vi "16 pulses TX.vi"(7 "reset system clock":bool, 9 "IQ_run":bool=TRUE, 10 "PDW input Valid":bool, 11 "array PDW":u64[](array[numeric])=[0, 0, 0, 0]) -> (0 "dds free":bool[](array[boolean]), 1 "fpga clock":u64, 2 "output valid":bool, 3 "RF OUT":T1, 4 "ready for input":bool, 5 "pulse transmitted":u32)   [LabVIEW 2021]
uses:
  <instrlib>/_niInstr/DSP/v1/Shared/Public/IQ Data.ctl
  <instrlib>/_niInstr/Basic Elements/v1/FPGA/Private/Count Up U64.vi
  <instrlib>/_niInstr/Basic Elements/v1/FPGA/Private/Count Up U32.vi
  <instrlib>/_niInstr/Basic Elements/v1/FPGA/niInstr Basic Elements v1 FPGA.lvlib
  <instrlib>/_niInstr/DSP/v1/Shared/niInstr DSP v1 Shared.lvlib
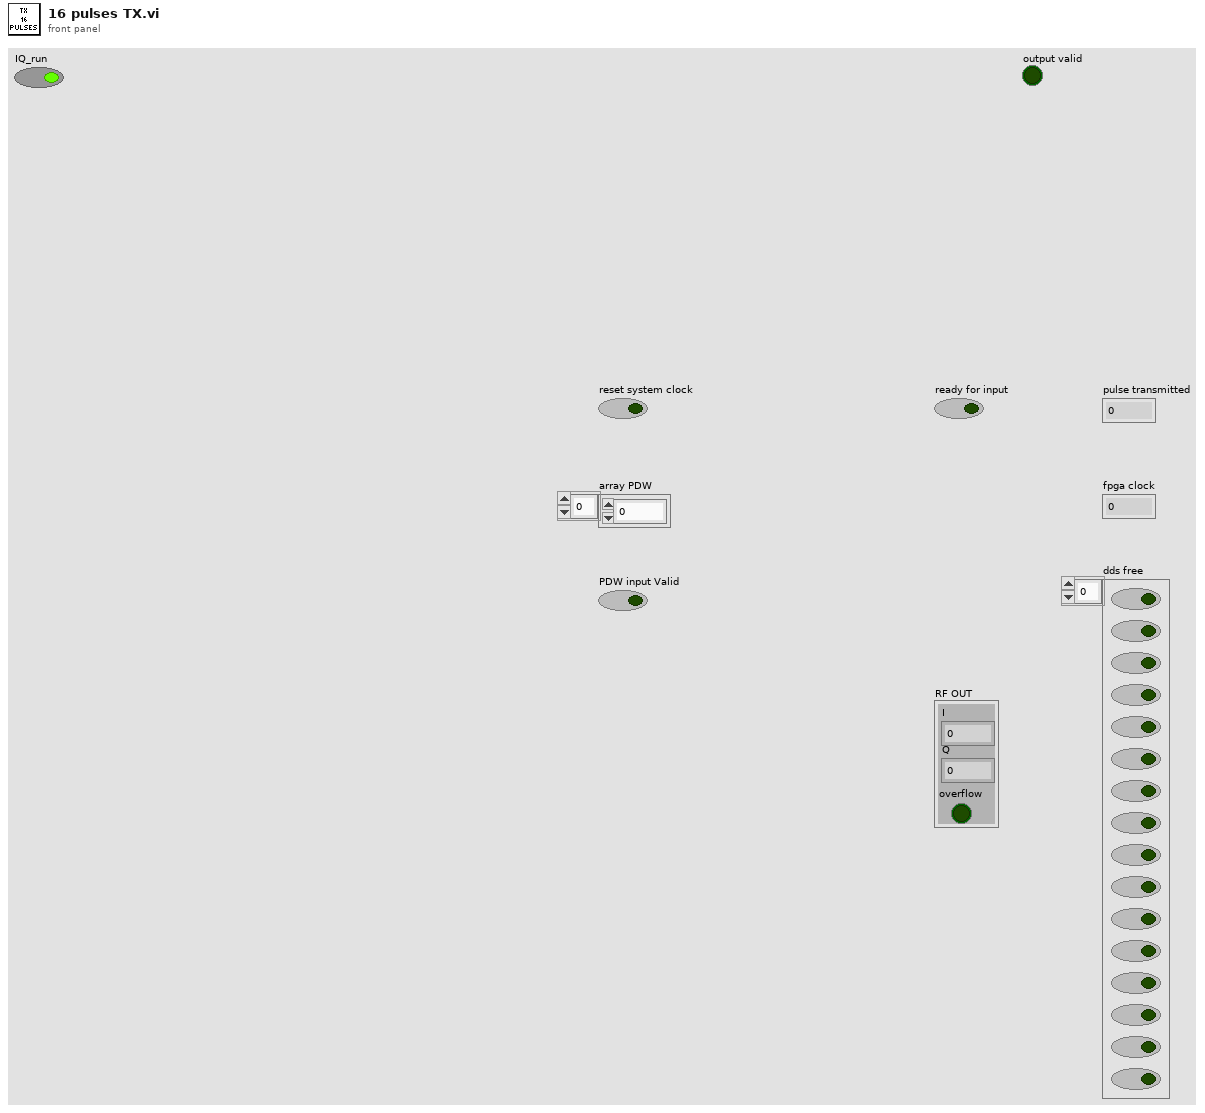
[diagram p1: front panel]
types:
  T1 = typedef "niInstr DSP v1 Shared.lvlib/IQ Data.ctl" = cluster{"I":fxp<+/-,18,1>, "Q":fxp<+/-,18,1>, "overflow":bool}
  T2 = typedef "pdw.ctl" = cluster{"PW":u32, "frequency shift":fxp<+/-,48,0>, "amp":fxp<+/-,18,1>, "mode type":T3, "mode depth":u32, "mode filter":u8}
  T3 = typedef "mode_type.ctl" = enum8{"CW", "NC - CW", "NC - cw", "LFM", "BPSK", "QPSK"}
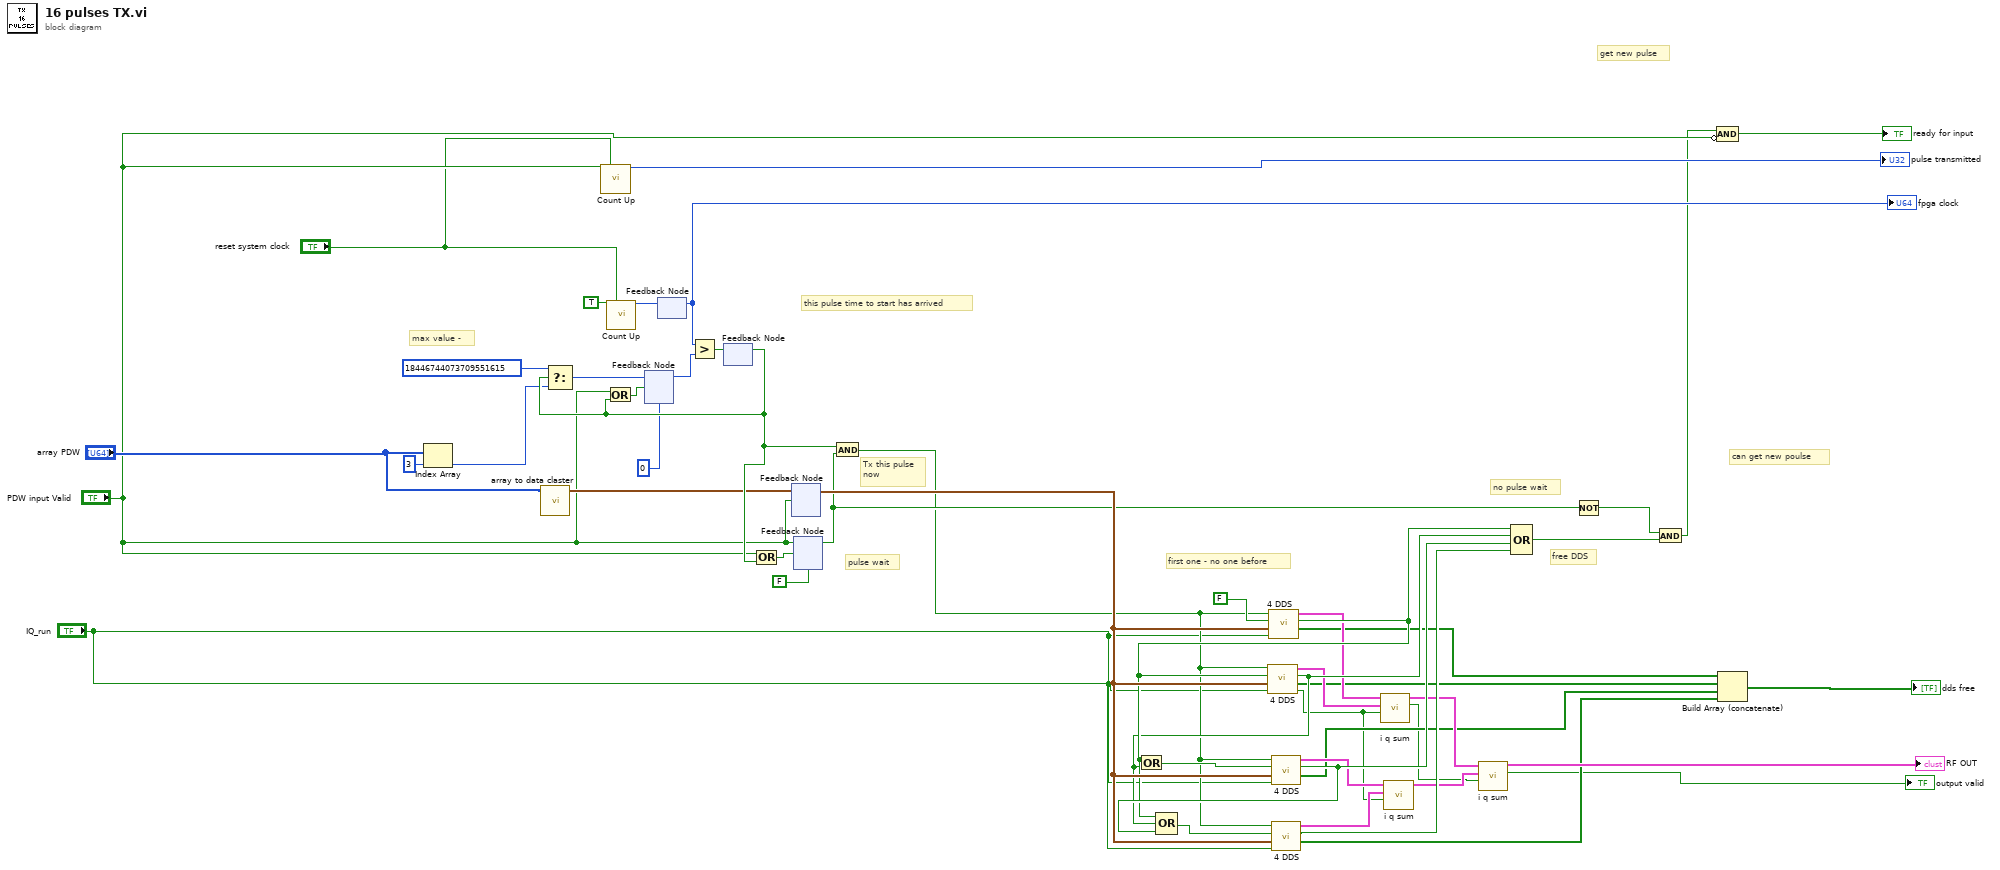
[diagram p0: block diagram]
diagram:
  # "this pulse time to start has arrived"
  # "first one - no one before"
  # "max value -"
  # "Tx this pulse\nnow"
  # "get new pulse"
  # "pulse wait"
  # "can get new poulse"
  # "no pulse wait"
  # "free DDS"
  n1 = Index Array(array="array PDW", index=3) -> (element=w45:u64)
  n2 = call "array to data claster.vi"("Array"="array PDW") -> ("Cluster"=w26:T2)  [unwired: 10 in]
  n3 = call-poly <instrlib>:"Count Up.vi"("increment"="PDW input Valid", "reset"="reset system clock") -> ("count out"=→"pulse transmitted":u32)  [unwired: 13 in]
  n4 = call-poly <instrlib>:"Count Up.vi"("increment"=TRUE, "reset"="reset system clock") -> ("count out"=w24:u64)  [unwired: 13 in]
  n5 = feedback #1(u64 0 ("U64")) -> (w11:u64)
  n6 = feedback #2() -> (w25:u64)  [unwired: 1 in]
  "fpga clock" <- w25
  n7 = feedback-in #2(w24) -> ()
  n8 = Greater?(x=w25, y=w11) -> (0:w48:bool)
  n9 = feedback #3() -> (w49:bool)  [unwired: 1 in]
  n10 = Select(t=u64 18446744073709551615, s=w49, f=w45) -> (s? t:f=w16:u64)
  n11 = Or(x="PDW input Valid", y=w49) -> (x .or. y?=w17:bool)
  n12 = feedback-in #1(w16, w17) -> ()
  n13 = feedback-in #3(w48) -> ()
  n14 = Or(x="PDW input Valid", y=w49) -> (x .or. y?=w22:bool)
  n15 = feedback #4() -> (w42:T2)  [unwired: 1 in]
  n16 = feedback-in #4(w26, "PDW input Valid") -> ()
  n17 = feedback #5(FALSE ("Output Valid")) -> (w34:bool)
  n18 = feedback-in #5("PDW input Valid", w22) -> ()
  n19 = And(x=w49, y=w34) -> (x .and. y?=w9:bool)
  n20 = call "4 DDS.vi"("input valid"="IQ_run", "pdw in"=w42, "free DDS before me?"=FALSE, "new PDW in"=w9) -> ("state of every DDS"=w8:bool[], "have free DDS"=w40:bool, "IQ out"=w33:T1)  [unwired: 4 in, 1 out]
  n21 = call "4 DDS.vi"("input valid"="IQ_run", "pdw in"=w42, "free DDS before me?"=w40, "new PDW in"=w9) -> ("output valid"=w3:bool, "state of every DDS"=w7:bool[], "have free DDS"=w39:bool, "IQ out"=w35:T1)  [unwired: 4 in]
  n22 = Or(x=w40, y=w39) -> (x .or. y?=w36:bool)
  n23 = call "4 DDS.vi"("input valid"="IQ_run", "pdw in"=w42, "free DDS before me?"=w36, "new PDW in"=w9) -> ("state of every DDS"=w6:bool[], "have free DDS"=w43:bool, "IQ out"=w37:T1)  [unwired: 4 in, 1 out]
  n24 = Compound Arithmetic op=OR(w40, w39, w43) -> (w41:bool)
  n25 = call "4 DDS.vi"("input valid"="IQ_run", "pdw in"=w42, "free DDS before me?"=w41, "new PDW in"=w9) -> ("state of every DDS"=w5:bool[], "have free DDS"=w44:bool, "IQ out"=w38:T1)  [unwired: 4 in, 1 out]
  n26 = call "i q sum.vi"("input valid"=w3, 10:"data in"=w35, 11:"data in"=w33) -> ("output valid"=w2:bool, "output cluster"=w29:T1)  [unwired: 7 in]
  n27 = call "i q sum.vi"("input valid"=w3, 10:"data in"=w38, 11:"data in"=w37) -> ("output cluster"=w31:T1)  [unwired: 7 in, 1 out]
  n28 = call "i q sum.vi"("input valid"=w2, 10:"data in"=w31, 11:"data in"=w29) -> ("output valid"=→"output valid":bool, "output cluster"=→"RF OUT":T1)  [unwired: 7 in]
  n29 = Compound Arithmetic op=OR(w40, w39, w43, w44) -> (w27:bool)
  n30 = Not(x=w34) -> (.not. x?=w12:bool)
  n31 = And(x=w12, y=w27) -> (x .and. y?=w13:bool)
  n32 = Compound Arithmetic op=AND(w13, invert "PDW input Valid") -> (→"ready for input":bool)
  n33 = Build Array (concatenate)(w8, w7, w6, w5) -> (→"dds free":bool[])
